vi "Create Upload Initiate Response Message.vi"(11 "Service Data Object in":refnum<class "Service Data Object.lvclass">) -> (2 "Response Message":refnum<class "CANopen Message.lvclass">, 3 "Service Data Object out":refnum<class "Service Data Object.lvclass">)   [LabVIEW 2024, in "Service Data Object.lvclass"]
uses:
  Service Data Object.lvclass
  CANopen Message/CANopen Message.lvclass
  CANopen/FunctionCode.ctl
  Service Data Object.lvclass/Service Data Object.ctl
  CANopen Master.lvlib
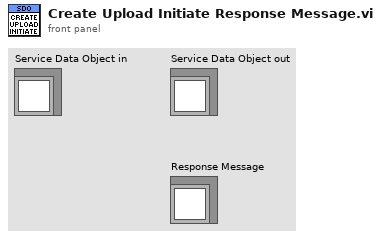
[diagram p1: front panel]
types:
  T1 = typedef "CANopen Master.lvlib/FunctionCode.ctl" = u16
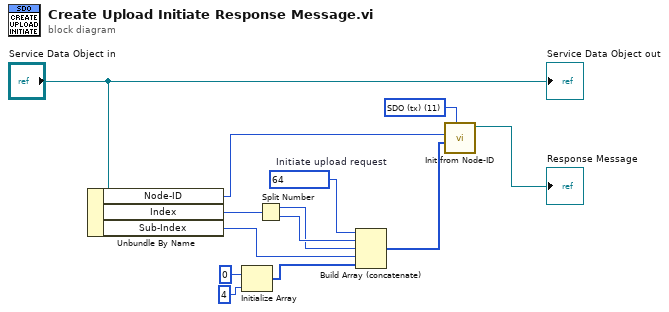
[diagram p0: block diagram]
diagram:
  w6 = u8 64  # Initiate upload request
  w12 = T1 11 items=["EMCY"=1, "PDO1 (tx)"=3, "PDO1 (rx)"=4, "PDO2 (tx)"=5, "PDO2 (rx)"=6, "PDO3 (tx)"=7, "PDO3 (rx)"=8, "PDO4 (tx)"=9, "PDO4 (rx)"=10, "SDO (tx)"=11, "SDO (rx)"=12, "NMT error control"=14] ("Function code")
  n1 = Unbundle By Name("Service Data Object in") -> ("Node-ID"=w3:u8, "Index"=w5:u16, "Sub-Index"=w4:u8)
  n2 = Initialize Array(u8 0, 4 ("y")) -> (w8:u8[])
  n3 = Split Number(x=w5) -> (hi(x)=w10:u8, lo(x)=w11:u8)
  n4 = Build Array (concatenate)(w6, w11, w10, w4, w8) -> (w2:u8[])
  n5 = call "Init from Node-ID.vi"("Function code"=w12, "Data"=w2, "Node-ID"=w3) -> ("CANopen Message out"=→"Response Message":refnum<class "CANopen Message.lvclass">)  [unwired: 8 in]
  "Service Data Object out" <- "Service Data Object in"
